vi "DAQ Application.vi"() -> ()   [LabVIEW 2025]
panel:
  in  "Amplitude":dbl=1.0
  in  "Frequency":dbl=10.1
  in  "Offset":dbl
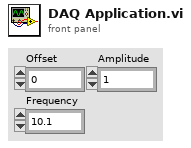
[diagram p1: front panel]
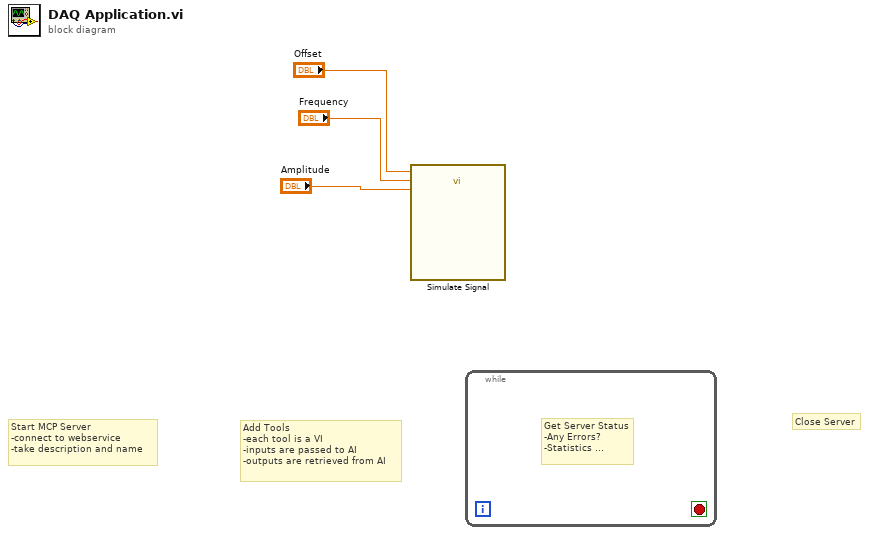
[diagram p0: block diagram]
diagram:
  # "Close Server"
  # "Add Tools\n-each tool is a VI\n-inputs are passed to AI\n-outputs are retrieved from AI"
  # "Start MCP Server\n-connect to webservice\n-take description and name"
  n1 = call "Simulate Signal"("Offset"="Offset", "Frequency"="Frequency", "Amplitude"="Amplitude") -> ()  [unwired: 11 in, 2 out]
  n2 = while {
    stop <- _ stop-if-true
    # "Get Server Status\n-Any Errors?\n-Statistics ..."
  }
